vi "波形图标（多条曲线）.vi"() -> ()   [LabVIEW 2017]
panel:
  out "波形图表":cluster{dbl, dbl}(graph)
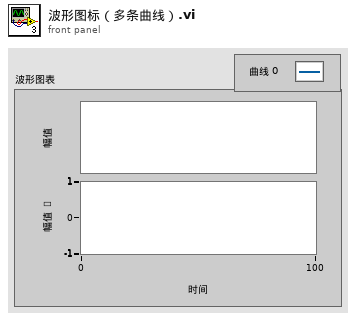
[diagram p1: front panel]
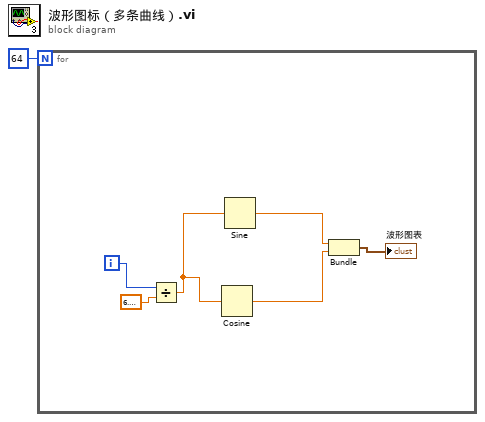
[diagram p0: block diagram]
diagram:
  n1 = for {
    N: 64 -> [_]
    i -> [w6]
    n2 = Divide(x=w6, y=6.283185307179586) -> (x/y=w5:dbl)
    n3 = Cosine(x=w5) -> (cos(x)=w3:dbl)
    n4 = Sine(x=w5) -> (sin(x)=w4:dbl)
    n5 = Bundle(w4, w3) -> (→"波形图表":cluster{dbl, dbl})  [unwired: 1 in]
  }
